vi "Begin.vi"(8 "error in":errorcluster) -> (0 "error out":errorcluster)   [LabVIEW 2016]
doc: "Called before other user functions, this VI is expected to open initial I/O refnums, load in file data, and do all program initialization. Notice that the <B>error out</B> terminal is simply used for data flow. Wiring it to other structures or subVIs ensures that this VI runs first."
uses:
  <vilib>/Rock Robotics/WPI/DriverStation/WPI_DriverStationRobotMode2.ctl
  <vilib>/Rock Robotics/WPI/Joystick/WPI_JoystickDeviceEnum.ctl
  <vilib>/Rock Robotics/WPI/ThirdParty/CanMotor/TalonSRX/WPI_CANTalonSRX_APIControlMode.ctl
  <vilib>/Rock Robotics/WPI/SafetyOutput/WPI_SafetyOutputConfigMenu.ctl
  <vilib>/Rock Robotics/SystemInterfaces/DIO/FPGA_DIOPWMChannel.ctl
  <vilib>/Rock Robotics/WPI/ThirdParty/CanMotor/TalonSRX/WPI_CANTalonSRX_APIFeedbackSelect.ctl
  <vilib>/Rock Robotics/WPI/Solenoid/WPI_SolenoidChannel.ctl
  <vilib>/Rock Robotics/WPI/Accelerometer/WPI_AccelerometerRange.ctl
  <vilib>/Rock Robotics/SystemInterfaces/AI/FPGA_AIGyroChannel.ctl
  <vilib>/Rock Robotics/SystemInterfaces/DIO/FPGA_DIOChannel.ctl
  Robot Global Data.vi
  <vilib>/Rock Robotics/Network Tables/NT Write String Array.vi
  <vilib>/Rock Robotics/WPI/MotorControl/WPI_MotorControlOpen VictorSP.vi
  <vilib>/Rock Robotics/WPI/Solenoid/WPI_SolenoidOpenDouble.vi
  <vilib>/Rock Robotics/WPI/Utilities/WPI_GetSetVariantRefNum.vi
  <vilib>/Rock Robotics/WPI/Accelerometer/InternalAccelerometer/WPI_AccelerometerInternalOpen.vi
  <vilib>/Rock Robotics/WPI/Gyro/WPI_GyroAnalogOpen.vi
  <vilib>/Rock Robotics/WPI/Ultrasonic/WPI_SonarSRF04DigitalOpen.vi
  <vilib>/Rock Robotics/WPI/Ultrasonic/WPI_SonarSRF04DigitalRefNum Registry Set.vi
  <vilib>/Rock Robotics/WPI/Counter/WPI_CounterDigitalInputToDigitalSource.vi
panel:
  out "Array":errorcluster[](array[cluster])
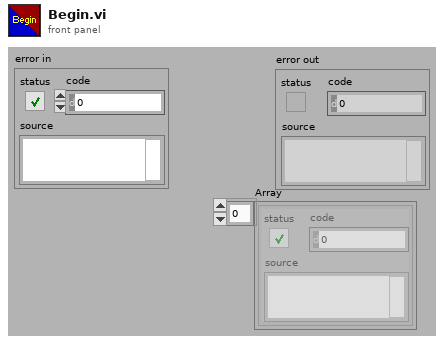
[diagram p1: front panel]
types:
  T1 = typedef "WPI_DriverStationRobotMode2.ctl" = enum16{"Autonomous Disabled", "Autonomous Enabled", "Teleop Disabled", "Teleop Enabled", "Disconnected", "Finish", "Test Disabled", "Test Enabled", "Emergency Stopped"}
  T2 = typedef "WPI_JoystickDeviceEnum.ctl" = enum16{"USB 0", "USB 1", "USB 2", "USB 3", "USB 4", "USB 5"}
  T3 = typedef "FPGA_DIOPWMChannel.ctl" = enum8{"PWM 0", "PWM 1", "PWM 2", "PWM 3", "PWM 4", "PWM 5", "PWM 6", "PWM 7", "PWM 8", "PWM 9", "PWM MXP 0", "PWM MXP 1", "PWM MXP 2", "PWM MXP 3", "PWM MXP 4", "PWM MXP 5", "PWM MXP 6", "PWM MXP 7", "PWM MXP 8", "PWM MXP 9", "Invalid"}
  T4 = typedef "WPI_SafetyOutputConfigMenu.ctl" = enum16{"Enable", "Disable"}
  T5 = typedef "WPI_CANTalonSRX_APIFeedbackSelect.ctl" = enum16{"Digital Quadrature Encoder", "Analog Potentiometer", "Analog Encoder", "Count on Quad-A (Rising-Edge)", "Count on Quad-A (Falling-Edge)", "CTR Magnetic Enc (Absolute)", "CTR Magnetic Enc (Relative)", "Pulse Width"}
  T6 = typedef "WPI_CANTalonSRX_APIControlMode.ctl" = enum8{"Percent VBus", "Speed", "Position", "Slave", "Unchanged / Invalid", "Voltage Compensation", "Current", "Motion Profile", "Motion Magic"}
  T7 = typedef "WPI_SolenoidChannel.ctl" = enum8{"Solenoid 0", "Solenoid 1", "Solenoid 2", "Solenoid 3", "Solenoid 4", "Solenoid 5", "Solenoid 6", "Solenoid 7", "Invalid"}
  T8 = typedef "WPI_AccelerometerRange.ctl" = enum16{"+/- 2 g", "+/- 4 g", "+/- 8 g"}
  T9 = typedef "FPGA_AIGyroChannel.ctl" = enum8{"AI 0", "AI 1", "Invalid"}
  T10 = typedef "FPGA_DIOChannel.ctl" = enum8{"DIO 0", "DIO 1", "DIO 2", "DIO 3", "DIO 4", "DIO 5", "DIO 6", "DIO 7", "DIO 8", "DIO 9", "DIO MXP 0", "DIO MXP 1", "DIO MXP 2", "DIO MXP 3", "DIO MXP 4", "DIO MXP 5", "DIO MXP 6", "DIO MXP 7", "DIO MXP 8", "DIO MXP 9", "DIO MXP 10", "DIO MXP 11", "DIO MXP 12", "DIO MXP 13", "DIO MXP 14", "DIO MXP 15", "SPI Port CS1", "SPI Port CS2", "SPI Port CS3", "SPI Port MISO", "SPI Port MOSI", "Invalid"}
  T11 = typedef "WPI_JoystickDevRef.ctl" = cluster{"Device":T2}
  T12 = typedef "WPI_RobotDriveDevRef.ctl" = cluster{"DevStatus":errorcluster, "Motors[]":T13[], "Square Inputs":bool, "Max Output":dbl}
  T13 = typedef "WPI_MotorControlDeviceRef.ctl" = cluster{"DeviceStatus":errorcluster, "Type":T14, "PWM":cluster{"PWM Channel":T3, "DeadBand":T15}, "CAN":cluster{"Device Number":u8, "SetOutput VI Ref":variant, "GetOutput VI Ref":variant, "Enable VI Ref":variant, "Disable VI Ref":variant, "Data":variant}, "Invert":bool}
  T14 = typedef "WPI_MotorControlType.ctl" = enum16{"PWM", "CAN"}
  T15 = typedef "WPI_PWMDeadband.ctl" = cluster{"Name":string, "maxPositivePwm":i32, "minPositivePwm":i32, "centerPwm":i32, "maxNegativePwm":i32, "minNegativePwm":i32, "angularRange":u16}
  T16 = typedef "WPI_SolenoidDevRef.ctl" = cluster{"DevStatus":errorcluster, "Pneumatics Control Module":u8, "Forward Solenoid Channel":T7, "Reverse Solenoid Channel":T7}
  T17 = typedef "WPI_CompressorDevRef.ctl" = cluster{"DevStatus":errorcluster, "Pneumatics Control Module":u8}
  T18 = typedef "WPI_ServoDeviceRef.ctl" = cluster{"DeviceStatus":errorcluster, "PWM Channel":T3, "DeadBand":T15}
  T19 = typedef "WPI_AccelerometerDevRef.ctl" = cluster{"DevStatus":errorcluster, "Scaling":T20, "Analog Channels":T21, "I2C Bus":T23, "SPI Bus":T24, "Accel Range":T25, "ADXL Axes":T26, "Handle":i32, "Device Address":u8, "Accel Type":enum16{"Analog", "ADXL345 I2C", "ADXL345 SPI", "Internal", "ADXL362 SPI"}}
  T20 = typedef "WPI_AccelerometerScaling.ctl" = cluster{"Gain (VoltsPerG)":dbl, "Center Voltage":dbl}
  T21 = typedef "WPI_AccelerometerAnalogChannels.ctl" = cluster{"X-Axis":T22, "Y-Axis":T22, "Z-Axis":T22}
  T22 = typedef "FPGA_AIChannel.ctl" = enum8{"AI 0", "AI 1", "AI 2", "AI 3", "AI MXP 0", "AI MXP 1", "AI MXP 2", "AI MXP 3", "Invalid"}
  T23 = typedef "i2c_bus.ctl" = enum16{"I2C On-Board", "I2C MXP", "Invalid"}
  T24 = typedef "spi_bus.ctl" = enum16{"SPI On-Board, CS0", "SPI On-Board, CS1", "SPI On-Board, CS2", "SPI On-Board, CS3", "SPI MXP", "Invalid"}
  T25 = typedef "ADXL345 Range.ctl" = u8
  T26 = typedef "WPI_AccelerometerADXL345 Axes.ctl" = cluster{"X-Axis":bool, "Y-Axis":bool, "Z-Axis":bool}
  T27 = typedef "WPI_GyroDevRef.ctl" = cluster{"DevStatus":errorcluster, "Analog Channel":T22, "Offset":dbl, "Gain (VoltsPerDegree/Second)":dbl, "Gyro Type":enum16{"Analog", "XRS450"}, "Handle":i32, "SPI Bus":T24, "Device Found":bool, "Sample Rate":dbl, "Calibrate On Open":bool}
  T28 = typedef "WPI_DigitalInputDevRef.ctl" = cluster{"DevStatus":errorcluster, "DIO Channel":T10}
  T29 = typedef "FPGA_CounterEncoderSourceConvertionLVSourceType.ctl" = cluster{"DevStatus":errorcluster, "AnalogTriggerMode?":bool, "DigitalMode":cluster{"DIO Channel":T30}, "AnalogTriggerMode":cluster{"AnalogTriggerIndex":T31, "OutputType":T32}}
  T30 = typedef "FPGA_DIODigitalSourceChannel.ctl" = enum8{"DIO 0", "DIO 1", "DIO 2", "DIO 3", "DIO 4", "DIO 5", "DIO 6", "DIO 7", "DIO 8", "DIO 9", "DIO MXP 0", "DIO MXP 1", "DIO MXP 2", "DIO MXP 3", "DIO MXP 4", "DIO MXP 5", "DIO MXP 6", "DIO MXP 7", "DIO MXP 8", "DIO MXP 9", "DIO MXP 10", "DIO MXP 11", "DIO MXP 12", "DIO MXP 13", "DIO MXP 14", "DIO MXP 15", "Disabled"}
  T31 = typedef "FPGA_AnalogTriggerIndex.ctl" = enum8{"Trig 0", "Trig 1", "Trig 2", "Trig 3", "Trig 4", "Trig 5", "Trig 6", "Trig 7", "Invalid"}
  T32 = typedef "FPGA_AnalogTriggerOutType.ctl" = enum16{"InWindow", "TriggerState", "Rising", "Falling"}
  T33 = typedef "WPI_EncoderDevRef.ctl" = cluster{"DevStatus":errorcluster, "EncoderIndex":T34, "CounterIndex":T35, "DistancePerCount":dbl, "Decoding Type":T36}
  T34 = typedef "FPGA_EncoderIdx.ctl" = enum8{"Enc 0", "Enc 1", "Enc 2", "Enc 3", "Enc 4", "Enc 5", "Enc 6", "Enc 7", "Invalid"}
  T35 = typedef "FPGA_CounterCtrSystemIndex.ctl" = enum8{"Ctr 0", "Ctr 1", "Ctr 2", "Ctr 3", "Ctr 4", "Ctr 5", "Ctr 6", "Ctr 7", "Invalid"}
  T36 = typedef "WPI_EncoderType.ctl" = enum16{"1x", "2x", "4x"}
  T37 = typedef "WPI_UltrasonicDeviceRef.ctl" = cluster{"DevStatus":errorcluster, "Ping Channel":T10, "Echo Channel":T10, "CntIndex":T35}
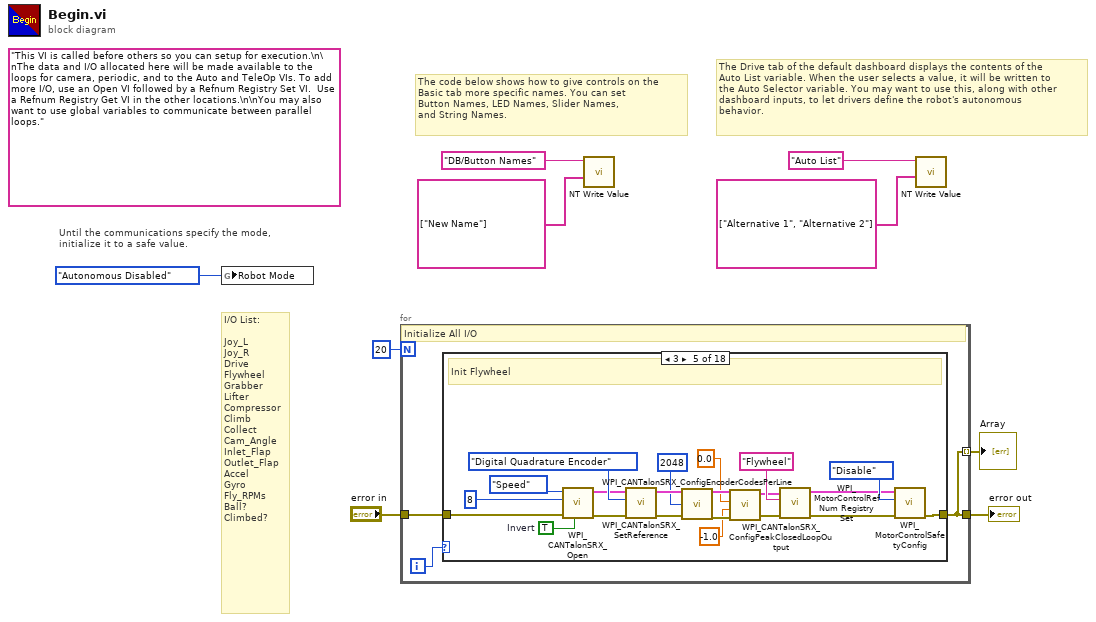
[diagram p0: block diagram]
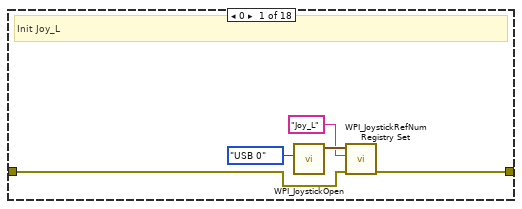
[diagram p2: hidden frame]
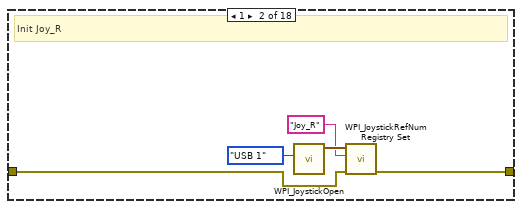
[diagram p3: hidden frame]
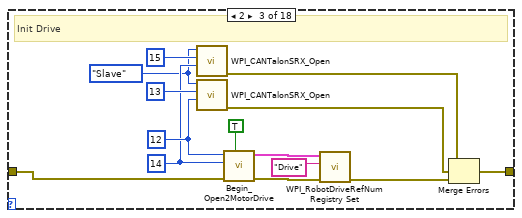
[diagram p4: hidden frame]
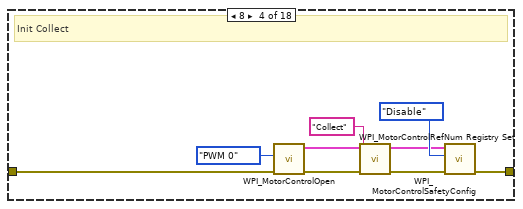
[diagram p5: hidden frame]
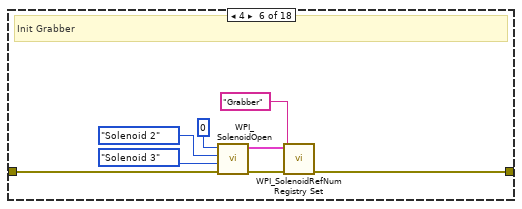
[diagram p6: hidden frame]
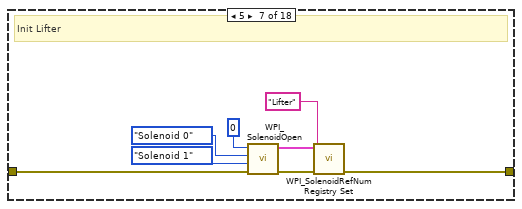
[diagram p7: hidden frame]
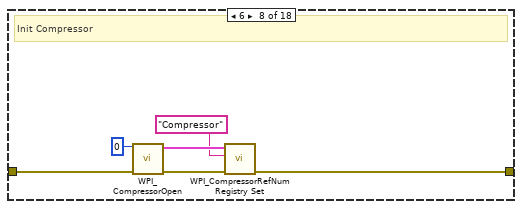
[diagram p8: hidden frame]
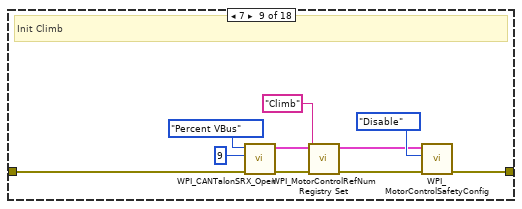
[diagram p9: hidden frame]
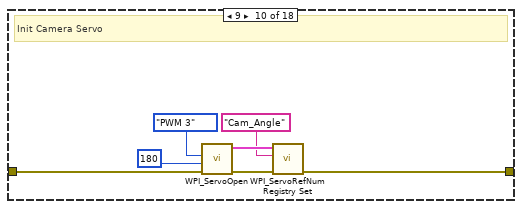
[diagram p10: hidden frame]
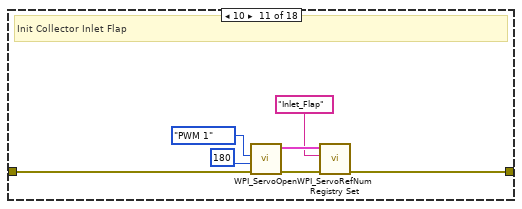
[diagram p11: hidden frame]
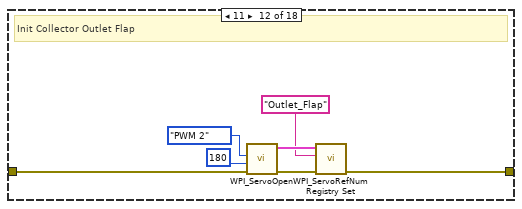
[diagram p12: hidden frame]
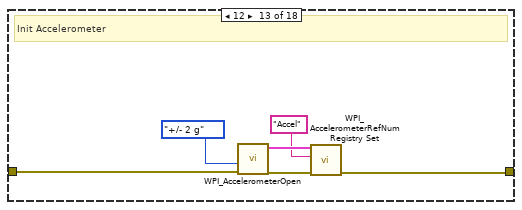
[diagram p13: hidden frame]
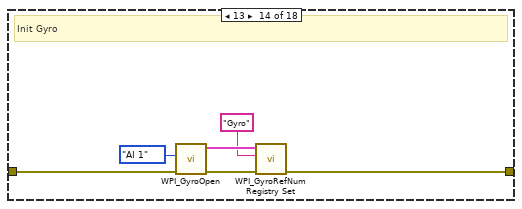
[diagram p14: hidden frame]
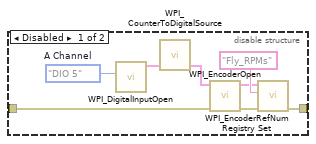
[diagram p16: hidden frame]
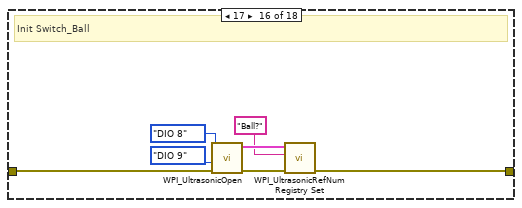
[diagram p17: hidden frame]
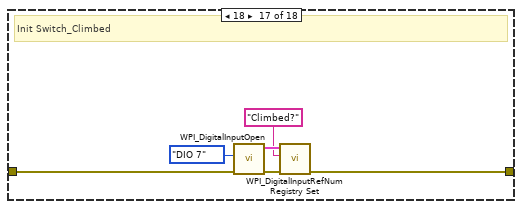
[diagram p18: hidden frame]
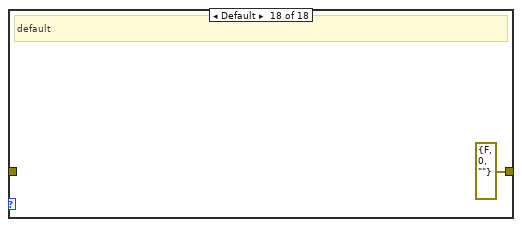
[diagram p19: hidden frame]
diagram:
  (unwired) "This VI is called before others so you can setup for execution.\n\nThe data and I/O allocated here will be made available to the loops for camera, periodic, and to the Auto and TeleOp VIs. To add more I/O, use an Open VI followed by a Refnum Registry Set VI.  Use a Refnum Registry Get VI in the other locations.\n\nYou may also want to use global variables to communicate between parallel loops."
  # "I/O List:\n\nJoy_L\nJoy_R\nDrive\nFlywheel\nGrabber\nLifter\nCompressor\nClimb\nCollect\nCam_Angle\nInlet_Flap\nOutlet_Flap\nAccel\nGyro\nFly_RPMs\nBall?\nClimbed?"
  # "The Drive tab of the default dashboard displays the contents of the\nAuto List variable. When the user selects a value, it will be written to\nthe Auto Selector variable. You may want to use this, along with other\ndashboard inputs, to let drivers define the robot's autonomous\nbehavior."
  # "The code below shows how to give controls on the\nBasic tab more specific names. You can set\nButton Names, LED Names, Slider Names,\nand String Names."
  # "Until the communications specify the mode,\ninitialize it to a safe value."
  n1 = global write "Robot Global Data.vi" "Robot Mode"(WPI_DriverStationRobotMode2."Autonomous Disabled" ("Robot Mode")) -> ()
  n2 = for {
    N: 20 -> [_]
    tunnel: [w10] -> w2
    tunnel: "error in" -> [w12]
    tunnel: [w10] -> w1 mode=indexing
    i -> [w11]
    # "Initialize All I/O"
    n3 = case shown="3" w11 {
      tunnel: [w15 w20 w27 w42 w63 w69 w76 w84 w90 w99 w106 w113 w120 w127 w133 w147 w150 errorcluster {"status"=FALSE, "code"=0, "source"=""} ("error out")] -> w10
      tunnel: w12 -> [w13 w18 w25 w38 w57 w72 w77 w87 w96 w104 w111 w114 w124 w131 w132 w146 w151 _]
      frame 0 {
        # "Init Joy_L"
        n4 = call <vilib>:"WPI_JoystickOpen.vi"("JoystickDevice"=WPI_JoystickDeviceEnum."USB 0") -> ("JoystickDevRef"=w16:T11)  [unwired: 10 in]
        n5 = call <vilib>:"WPI_JoystickRefNum Registry Set.vi"("error in (no error)"=w13, "refnum name"="Joy_L", "JoystickDevRef"=w16) -> ("error out"=w15:errorcluster)  [unwired: 7 in, 1 out]
      }
      frame 1 {
        # "Init Joy_R"
        n6 = call <vilib>:"WPI_JoystickOpen.vi"("JoystickDevice"=WPI_JoystickDeviceEnum."USB 1") -> ("JoystickDevRef"=w21:T11)  [unwired: 10 in]
        n7 = call <vilib>:"WPI_JoystickRefNum Registry Set.vi"("error in (no error)"=w18, "refnum name"="Joy_R", "JoystickDevRef"=w21) -> ("error out"=w20:errorcluster)  [unwired: 7 in, 1 out]
      }
      frame 2 {
        w26 = WPI_CANTalonSRX_APIControlMode."Slave" ("Control Mode")
        w30 = u8 14 ("Right Motor ID")
        w32 = u8 12 ("Left Motor ID")
        # "Init Drive"
        n8 = call <vilib>:"WPI_CANTalonSRX_Open.vi"("Master Device Number"=w30, "Device Number"=u8 15, "Control Mode"=w26) -> ("error out"=w24:errorcluster)  [unwired: 7 in, 1 out]
        n9 = call <vilib>:"WPI_CANTalonSRX_Open.vi"("Master Device Number"=w32, "Device Number"=u8 13, "Control Mode"=w26) -> ("error out"=w23:errorcluster)  [unwired: 7 in, 1 out]
        n10 = call "Begin_Open2MotorDrive.vi"("Left Motor Inverted"=TRUE, "error in (no error)"=w25, "Right Motor ID"=w30, "Left Motor ID"=w32) -> ("error out"=w33:errorcluster, "RobotDriveDevRef"=w35:T12)  [unwired: 6 in]
        n11 = call <vilib>:"WPI_RobotDriveRefNum Registry Set.vi"("error in (no error)"=w33, "refnum name"="Drive", "RobotDriveDevRef"=w35) -> ("error out"=w28:errorcluster)  [unwired: 7 in, 1 out]
        n12 = Merge Errors(w24, w23, w28) -> (w27:errorcluster)
      }
      frame 8 {
        # "Init Collect"
        n13 = call-poly <vilib>:"WPI_MotorControlOpen.vi"("error in (no error)"=w38, "PWM Channel"=FPGA_DIOPWMChannel."PWM 0") -> ("error out"=w39:errorcluster, "MotorControlDeviceRef"=w40:T13)  [unwired: 8 in]
        n14 = call <vilib>:"WPI_MotorControlRefNum Registry Set.vi"("error in (no error)"=w39, "refnum name"="Collect", "MotorControlDevRef"=w40) -> ("error out"=w43:errorcluster, "MotorControlDevRef"=w41:T13)  [unwired: 7 in]
        n15 = call <vilib>:"WPI_MotorControlSafetyConfig.vi"("error in (no error)"=w43, "mode"=WPI_SafetyOutputConfigMenu."Disable", "MotorControlDevRef"=w41) -> ("error out"=w42:errorcluster)  [unwired: 7 in, 1 out]
      }
      frame 3 {
        w52 = TRUE  # Invert
        # "Init Flywheel"
        n16 = call <vilib>:"WPI_CANTalonSRX_Open.vi"("Invert"=w52, "error in"=w57, "Device Number"=u8 8, "Control Mode"=WPI_CANTalonSRX_APIControlMode."Speed") -> ("error out"=w59:errorcluster, "CAN Talon SRX Ref"=w60:T13)  [unwired: 6 in]
        n17 = call <vilib>:"WPI_CANTalonSRX_SetReference.vi"("error in (no error)"=w59, "Feedback Reference"=WPI_CANTalonSRX_APIFeedbackSelect."Digital Quadrature Encoder", "CAN Talon SRX Ref"=w60) -> ("error out"=w54:errorcluster, "CAN Talon SRX Ref"=w55:T13)  [unwired: 7 in]
        n18 = call <vilib>:"WPI_CANTalonSRX_ConfigEncoderCodesPerLine.vi"("CAN Talon SRX Ref"=w55, "Number Encoder Lines\n(Counts Per Rotation)"=u32 2048 ("Number Encoder Lines\n(Counts Per Rotation)"), "error in (no error)"=w54) -> ("CAN Talon SRX Ref"=w50:T13, "error out"=w51:errorcluster)  [unwired: 11 in]
        n19 = call <vilib>:"WPI_CANTalonSRX_ConfigPeakClosedLoopOutput.vi"("error in (no error)"=w51, "Reverse Peak Output"=-1.0 ("Reverse Limit Position"), "Forward Peak Output"=0.0, "CAN Talon SRX Ref"=w50) -> ("error out"=w48:errorcluster, "CAN Talon SRX Ref"=w49:T13)  [unwired: 6 in]
        n20 = call <vilib>:"WPI_MotorControlRefNum Registry Set.vi"("error in (no error)"=w48, "refnum name"="Flywheel", "MotorControlDevRef"=w49) -> ("error out"=w66:errorcluster, "MotorControlDevRef"=w64:T13)  [unwired: 7 in]
        n21 = call <vilib>:"WPI_MotorControlSafetyConfig.vi"("error in (no error)"=w66, "mode"=WPI_SafetyOutputConfigMenu."Disable", "MotorControlDevRef"=w64) -> ("error out"=w63:errorcluster)  [unwired: 7 in, 1 out]
      }
      frame 4 {
        # "Init Grabber"
        n22 = call-poly <vilib>:"WPI_SolenoidOpen.vi"("error in (no error)"=w72, "Reverse Solenoid Channel"=WPI_SolenoidChannel."Solenoid 3" ("Solenoid Channel"), "Forward Solenoid Channel"=WPI_SolenoidChannel."Solenoid 2" ("Solenoid Channel"), "Pneumatics Control Module (0)"=u8 0) -> ("error out"=w70:errorcluster, "SolenoidDevRef"=w71:T16)  [unwired: 6 in]
        n23 = call <vilib>:"WPI_SolenoidRefNum Registry Set.vi"("error in (no error)"=w70, "refnum name"="Grabber", "SolenoidDevRef"=w71) -> ("error out"=w69:errorcluster)  [unwired: 7 in, 1 out]
      }
      frame 5 {
        # "Init Lifter"
        n24 = call-poly <vilib>:"WPI_SolenoidOpen.vi"("error in (no error)"=w77, "Reverse Solenoid Channel"=WPI_SolenoidChannel."Solenoid 1", "Forward Solenoid Channel"=WPI_SolenoidChannel."Solenoid 0" ("Solenoid Channel"), "Pneumatics Control Module (0)"=u8 0) -> ("error out"=w81:errorcluster, "SolenoidDevRef"=w80:T16)  [unwired: 6 in]
        n25 = call <vilib>:"WPI_SolenoidRefNum Registry Set.vi"("error in (no error)"=w81, "refnum name"="Lifter", "SolenoidDevRef"=w80) -> ("error out"=w76:errorcluster)  [unwired: 7 in, 1 out]
      }
      frame 6 {
        # "Init Compressor"
        n26 = call <vilib>:"WPI_CompressorOpen.vi"("Pneumatics Control Module (0)"=u8 0, "error in (no error)"=w87) -> ("CompressorDevRef"=w86:T17, "error out"=w85:errorcluster)  [unwired: 12 in]
        n27 = call <vilib>:"WPI_CompressorRefNum Registry Set.vi"("error in (no error)"=w85, "refnum name"="Compressor", "CompressorDevRef"=w86) -> ("error out"=w84:errorcluster)  [unwired: 7 in, 1 out]
      }
      frame 7 {
        # "Init Climb"
        n28 = call <vilib>:"WPI_CANTalonSRX_Open.vi"("error in"=w96, "Device Number"=u8 9, "Control Mode"=WPI_CANTalonSRX_APIControlMode."Percent VBus") -> ("error out"=w95:errorcluster, "CAN Talon SRX Ref"=w94:T13)  [unwired: 7 in]
        n29 = call <vilib>:"WPI_MotorControlRefNum Registry Set.vi"("error in (no error)"=w95, "refnum name"="Climb", "MotorControlDevRef"=w94) -> ("error out"=w91:errorcluster, "MotorControlDevRef"=w89:T13)  [unwired: 7 in]
        n30 = call <vilib>:"WPI_MotorControlSafetyConfig.vi"("error in (no error)"=w91, "mode"=WPI_SafetyOutputConfigMenu."Disable", "MotorControlDevRef"=w89) -> ("error out"=w90:errorcluster)  [unwired: 7 in, 1 out]
      }
      frame 9 {
        # "Init Camera Servo"
        n31 = call <vilib>:"WPI_ServoOpen.vi"("error in (no error)"=w104, "Angular Range"=u16 180, "PWM Channel"=FPGA_DIOPWMChannel."PWM 3") -> ("error out"=w100:errorcluster, "ServoDeviceRef"=w102:T18)  [unwired: 7 in]
        n32 = call <vilib>:"WPI_ServoRefNum Registry Set.vi"("error in (no error)"=w100, "refnum name"="Cam_Angle", "ServoDeviceRef"=w102) -> ("error out"=w99:errorcluster)  [unwired: 7 in, 1 out]
      }
      frame 10 {
        # "Init Collector Inlet Flap"
        n33 = call <vilib>:"WPI_ServoOpen.vi"("error in (no error)"=w111, "Angular Range"=u16 180, "PWM Channel"=FPGA_DIOPWMChannel."PWM 1") -> ("error out"=w107:errorcluster, "ServoDeviceRef"=w109:T18)  [unwired: 7 in]
        n34 = call <vilib>:"WPI_ServoRefNum Registry Set.vi"("error in (no error)"=w107, "refnum name"="Inlet_Flap", "ServoDeviceRef"=w109) -> ("error out"=w106:errorcluster)  [unwired: 7 in, 1 out]
      }
      frame 11 {
        # "Init Collector Outlet Flap"
        n35 = call <vilib>:"WPI_ServoOpen.vi"("error in (no error)"=w114, "Angular Range"=u16 180, "PWM Channel"=FPGA_DIOPWMChannel."PWM 2") -> ("error out"=w115:errorcluster, "ServoDeviceRef"=w117:T18)  [unwired: 7 in]
        n36 = call <vilib>:"WPI_ServoRefNum Registry Set.vi"("error in (no error)"=w115, "refnum name"="Outlet_Flap", "ServoDeviceRef"=w117) -> ("error out"=w113:errorcluster)  [unwired: 7 in, 1 out]
      }
      frame 12 {
        # "Init Accelerometer"
        n37 = call-poly <vilib>:"WPI_AccelerometerOpen.vi"("error in"=w124, "Accel Range"=WPI_AccelerometerRange."+/- 2 g") -> ("error out"=w121:errorcluster, "AccelerometerDevRef"=w123:T19)  [unwired: 8 in]
        n38 = call <vilib>:"WPI_AccelerometerRefNum Registry Set.vi"("error in (no error)"=w121, "refnum name"="Accel", "AccelerometerDevRef"=w123) -> ("error out"=w120:errorcluster)  [unwired: 7 in, 1 out]
      }
      frame 13 {
        # "Init Gyro"
        n39 = call-poly <vilib>:"WPI_GyroOpen.vi"("error in (no error)"=w131, "Analog Channel"=FPGA_AIGyroChannel."AI 1") -> ("error out"=w128:errorcluster, "GyroDevRef"=w129:T27)  [unwired: 7 in, 1 out]
        n40 = call <vilib>:"WPI_GyroRefNum Registry Set.vi"("error in (no error)"=w128, "refnum name"="Gyro", "GyroDevRef"=w129) -> ("error out"=w127:errorcluster)  [unwired: 7 in, 1 out]
      }
      frame 16 {
        # "Init Fly_RPMs"
        n41 = disable-structure shown="Enabled" {
          disable-tunnel: [w135 w142] -> w133
          disable-tunnel: w132 -> [w134 w142]
          frame Disabled {
            w136 = FPGA_DIOChannel."DIO 5"  # A Channel
            n42 = call <vilib>:"WPI_DigitalInputOpen.vi"("DIO Channel"=w136) -> ("DigitalInputDevRef"=w137:T28)  [unwired: 1 in, 9 out]
            n43 = call-poly <vilib>:"WPI_CounterToDigitalSource.vi"("DigitalInputDevRef"=w137) -> ("Digital Source"=w138:T29)  [unwired: 6 out]
            n44 = call <vilib>:"WPI_EncoderOpen.vi"("error in (no error)"=w134, "ASource"=w138) -> ("error out"=w139:errorcluster, "EncoderDevRef"=w140:T33)  [unwired: 6 in, 2 out]
            n45 = call <vilib>:"WPI_EncoderRefNum Registry Set.vi"("error in (no error)"=w139, "refnum name"="Fly_RPMs", "EncoderDevRef"=w140) -> ("error out"=w135:errorcluster)  [unwired: 7 in, 1 out]
          }
          frame Enabled {
          }
        }
      }
      frame 17 {
        # "Init Switch_Ball"
        n46 = call-poly <vilib>:"WPI_UltrasonicOpen.vi"("error in (no error)"=w146, "Echo DIO Channel"=FPGA_DIOChannel."DIO 9", "Ping DIO Channel"=FPGA_DIOChannel."DIO 8") -> ("error out"=w149:errorcluster, "SonarSRF04DevRef"=w148:T37)  [unwired: 7 in]
        n47 = call-poly <vilib>:"WPI_UltrasonicRefNum Registry Set.vi"("error in (no error)"=w149, "refnum name"="Ball?", "SonarSRF04DevRef"=w148) -> ("error out"=w147:errorcluster)  [unwired: 7 in, 1 out]
      }
      frame 18 {
        # "Init Switch_Climbed"
        n48 = call <vilib>:"WPI_DigitalInputOpen.vi"("error in (no error)"=w151, "DIO Channel"=FPGA_DIOChannel."DIO 7") -> ("error out"=w154:errorcluster, "DigitalInputDevRef"=w153:T28)  [unwired: 8 in]
        n49 = call <vilib>:"WPI_DigitalInputRefNum Registry Set.vi"("error in (no error)"=w154, "refnum name"="Climbed?", "DigitalInputDevRef"=w153) -> ("error out"=w150:errorcluster)  [unwired: 7 in, 1 out]
      }
      frame Default {
        # "default"
      }
    }
  }
  "error out" <- w2
  "Array" <- w1
  n50 = call-poly <vilib>:"NT Write Value.vi"("String Array"=string[] ["New Name"], "Name"="DB/Button Names") -> ()  [unwired: 9 in, 1 out]
  n51 = call-poly <vilib>:"NT Write Value.vi"("String Array"=string[] ["Alternative 1", "Alternative 2"], "Name"="Auto List") -> ()  [unwired: 9 in, 1 out]
